vi "Read Worker.vi"(8 "error in (no error)":errorcluster, 11 "Worker Test in":refnum<class "Worker Test.lvclass">) -> (0 "error out":errorcluster, 2 "Worker":refnum<class "Worker.lvclass">, 3 "Worker Test out":refnum<class "Worker Test.lvclass">)   [LabVIEW 2020, in "Worker Test.lvclass"]
uses:
  Worker Test.lvclass
  C:/Program Files (x86)/National Instruments/LabVIEW 2020/vi.lib/Asteme/Triarc Framework Test Suite/Base Class Test/Base Test.lvclass
  Processes/People/Workers/Worker/Worker.lvclass
  <vilib>/Asteme/Triarc Framework Test Suite/Base Class Test/Base Test.lvclass/Base Test.ctl
  <vilib>/Asteme/Triarc Framework/Base/Base.lvclass
  <vilib>/Asteme/Triarc Framework Test Suite/Base Class Test/Base Test.lvclass
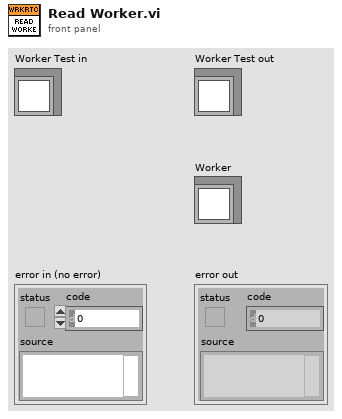
[diagram p1: front panel]
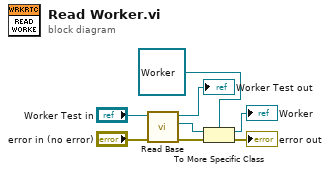
[diagram p0: block diagram]
diagram:
  n1 = call <vilib>:"Read Base.vi"("error in (no error)"="error in (no error)", "Base Class Test In"="Worker Test in") -> ("error out"=w8:errorcluster, "Base.lvclass"=w7:refnum<class "Base.lvclass">, "Base Class Test Out"=→"Worker Test out":refnum<class "Worker Test.lvclass">)  [unwired: 7 in]
  n2 = To More Specific Class(target class=refnum<class "Worker.lvclass"> refnum ("Worker.lvclass"), reference=w7, error in=w8) -> (specific class reference=→"Worker":refnum<class "Worker.lvclass">, error out=→"error out":errorcluster)
